vi "Calculate Tardiness (FIFO Engine).vi"(6 "Number of Machines":i32=4, 7 "Number of Jobs":i32=4, 9 "Due Dates":u16[](array[numeric]), 10 "Processing Times":u16[][](array[numeric]), 11 "Schedule In":u16[](array[numeric])) -> (3 "Tardiness(FIFO Engine)":u16)   [LabVIEW 2013, in "Scheduler.lvclass"]
uses:
  Scheduler.lvclass
  Scheduler_Class/Check Other Machines for Schedule Time.vi
  Scheduler_Class/Schedule Job.vi
  Scheduler_Class/Find Gaps on Particular Machine.vi
  Scheduler_Class/Increment Number of Jobs on Machine.vi
  Scheduler_Class/Operation to Machine Job Tuple.vi
  Scheduler_Class/Find Job On Other Machines.vi
panel:
  out "Job Completion Times":u16[](array[numeric])
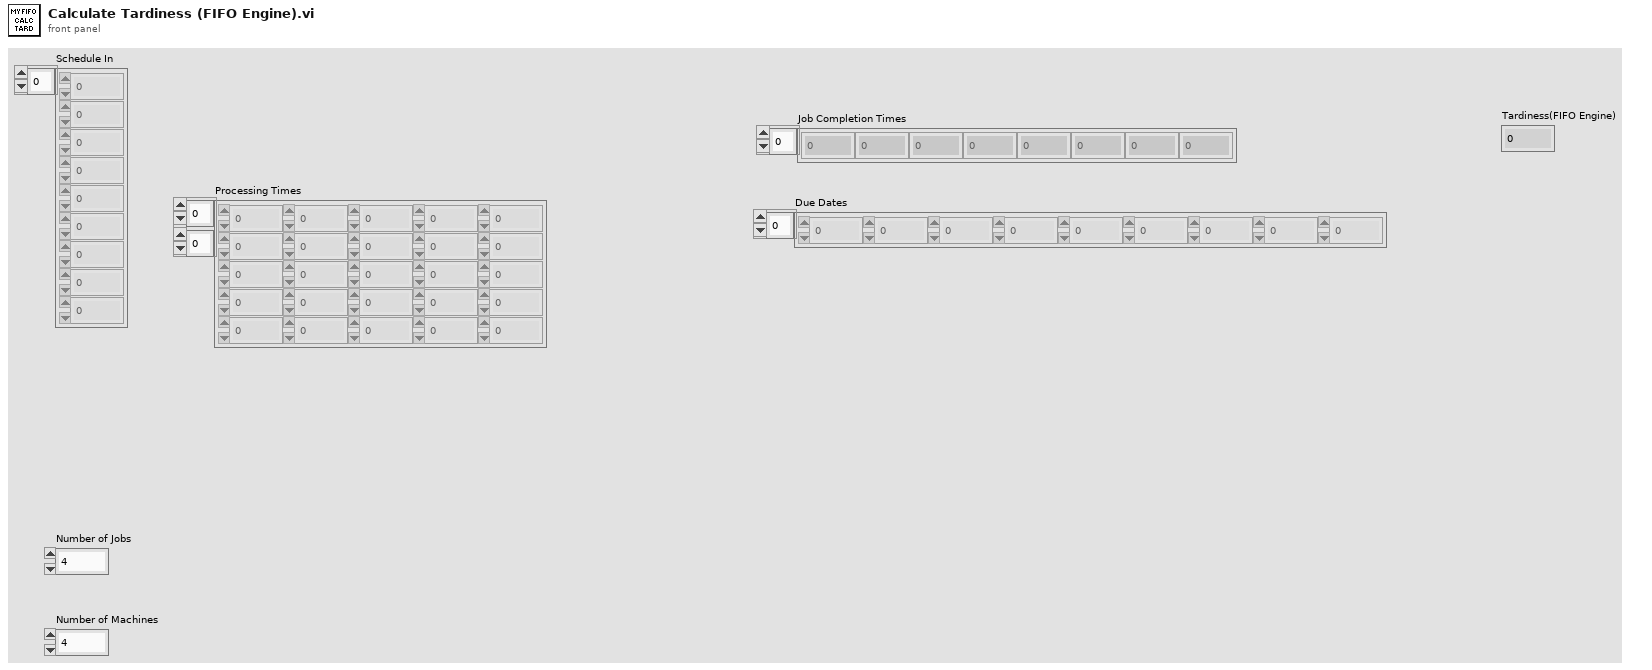
[diagram p1: front panel]
types:
  T1 = typedef "GanntChart_Element.ctl" = cluster{"Operation Number":i32, "Job Number":i32, "Start Time":i32, "Procesing Time":u16, "End Time":i32}
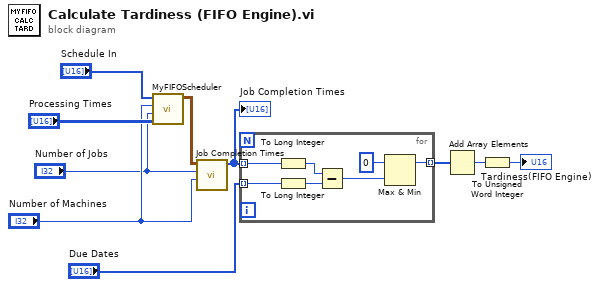
[diagram p0: block diagram]
diagram:
  n1 = call "MyFIFOScheduler.vi"("Processing Times (Rows Mach.Cols Jobs)"="Processing Times", "Number of Jobs"="Number of Jobs", "Number of Machines"="Number of Machines", "Schedule"="Schedule In") -> ("Gannt Chart Out"=w9:T1[][])  [unwired: 6 in, 1 out]
  n2 = call "Job Completion Times.vi"("Number Of Machines"="Number of Machines", "Number Of Jobs"="Number of Jobs", "Gannt Chart In"=w9) -> ("Job Completion Times"=w8:u16[])  [unwired: 8 in]
  "Job Completion Times" <- w8
  n3 = for {
    tunnel: "Due Dates" -> [w16] mode=indexing
    tunnel: w8 -> [w17] mode=indexing
    tunnel: [w11] -> w7 mode=indexing
    n4 = To Long Integer(number=w17) -> (32bit integer=w14:i32)
    n5 = To Long Integer(number=w16) -> (32bit integer=w15:i32)
    n6 = Subtract(x=w14, y=w15) -> (x-y=w13:i32)
    n7 = Max & Min(x=0, y=w13) -> (max(x,y)=w11:i32)  [unwired: 1 out]
  }
  n8 = Add Array Elements(numeric array=w7) -> (sum=w6:i32)
  n9 = To Unsigned Word Integer(number=w6) -> (unsigned 16bit integer=→"Tardiness(FIFO Engine)":u16)
